vi "FormatNotification.vi"(2 "Param in variant form":variant, 3 "message":string) -> (0 "Notification":variant)   [LabVIEW 2020]
uses:
  _controls/Notifier Cluster.ctl
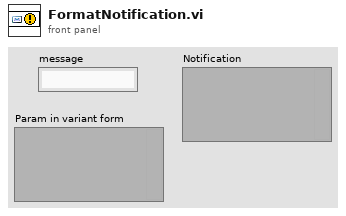
[diagram p1: front panel]
types:
  T1 = typedef "Notifier Cluster.ctl" = cluster{"message":string, "data":variant}
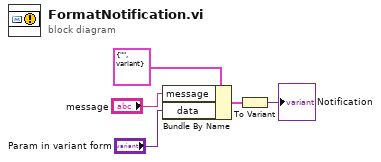
[diagram p0: block diagram]
diagram:
  n1 = Bundle By Name(cluster=T1 {"message"="", "data"=variant}, "message"="message", "data"="Param in variant form") -> (w4:T1)
  n2 = To Variant(anything=w4) -> (Variant=→"Notification":variant)
